vi "Tag Check.vi"(0 "Tree Reference In":refnum<vi>, 2 "Input Tag":string, 5 "error in (no error)":errorcluster) -> (14 "Tree Reference Out":refnum<vi>, 16 "Duplicate Tag":string, 17 "Tag OK":bool, 19 "error out":errorcluster)   [LabVIEW 2011, in "VITesterUtilities.lvlib"]
doc: "Checks the input tag and makes sure that it is a valid tag within the referenced tree. Returns all errors including the invalid tag error."
uses:
  Libraries/VITesterUtilities.lvlib
panel:
  # "VI INPUTS"
  # "VI OUTPUTS"
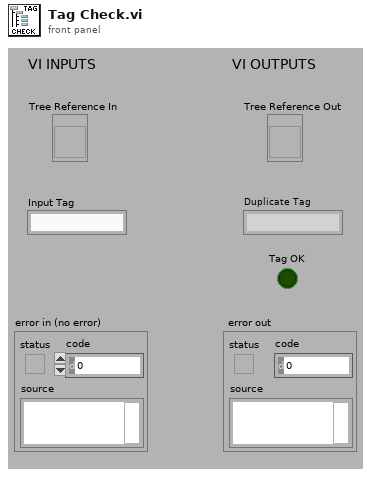
[diagram p1: front panel]
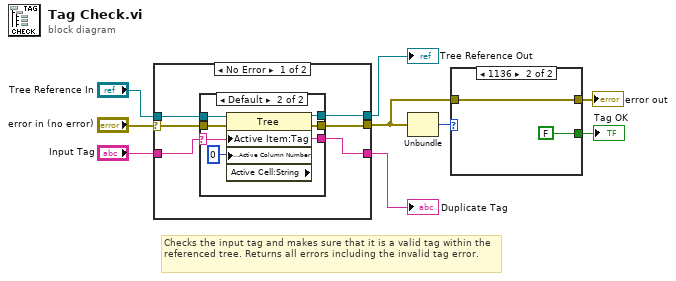
[diagram p0: block diagram]
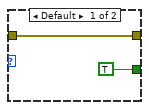
[diagram p2: hidden frame]
diagram:
  # "Checks the input tag and makes sure that it is a valid tag within the referenced tree. Returns all errors including the invalid tag error."
  n1 = case shown="No Error" "error in (no error)" {
    tunnel: "Tree Reference In" -> [w15 w27]
    selector: "error in (no error)" -> [w14 w26]
    tunnel: [w12 w27] -> w9
    tunnel: [w13 w26] -> w3
    tunnel: [w10 w25] -> w5
    tunnel: "Input Tag" -> [w11 w25]
    frame No Error {
      n2 = case shown="Default" w11 {
        selector: w11 -> [w16 w19]
        tunnel: w15 -> [w17 w24]
        tunnel: w14 -> [w18 w23]
        tunnel: [w18 w21] -> w13
        tunnel: [w17 w20] -> w12
        tunnel: [w16 w19] -> w10
        frame "" {
        }
        frame Default {
          n3 = property class="Tree" props=["Active Item:Tag", "Active Cell:Active Column Number", "Active Cell:String"](reference=w24, error in=w23, "Active Item:Tag"=w19, "Active Cell:Active Column Number"=0 ("Active Cell Properties:Active Column Number")) -> (reference out=w20:refnum<vi>, error out=w21:errorcluster)  [unwired: 1 out]
        }
      }
    }
    frame Error {
    }
  }
  "Tree Reference Out" <- w9
  "Duplicate Tag" <- w5
  n4 = Unbundle(w3) -> ("code"=w4:i32)  [unwired: 2 out]
  n5 = case shown="1136" w4 {
    tunnel: w3 -> [w29 w30]
    tunnel: [w29 w30] -> w2
    tunnel: [TRUE FALSE] -> w1
    frame Default {
    }
    frame 1136 {
    }
  }
  "error out" <- w2
  "Tag OK" <- w1
